vi "Initialize-parameter-refs.vi"(8 "error in (no error)":errorcluster, 11 "Data ref. in":refnum<data-value>) -> (0 "error out":errorcluster, 3 "Data ref.":refnum<data-value>)   [LabVIEW 2013, in "CameraVision.lvlib" / "CV-Main.lvclass"]
uses:
  CV-Main.lvclass
  CV-Main.lvclass/CV-Main.ctl
  Acquisition/CV-Acquisition.lvclass
  Analysis/CV-Analysis.lvclass
  Configuration/CV-Configuration.lvclass
  Correction/CV-Correction.lvclass
  Mapping/CV-Mapping.lvclass
  Storage/CV-Storage.lvclass
  Temperature/CV-Temperature.lvclass
  Filter/CV-Filter.lvclass
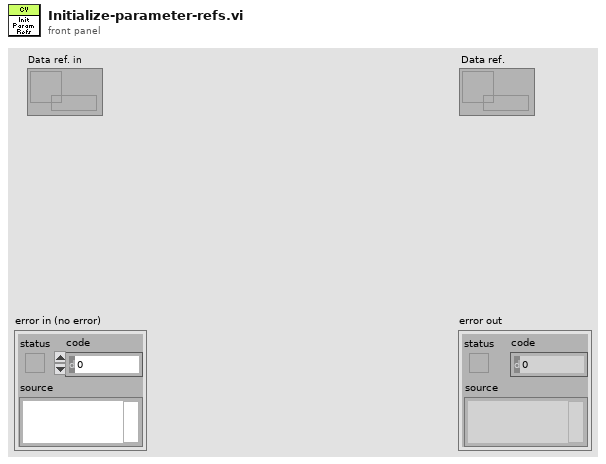
[diagram p1: front panel]
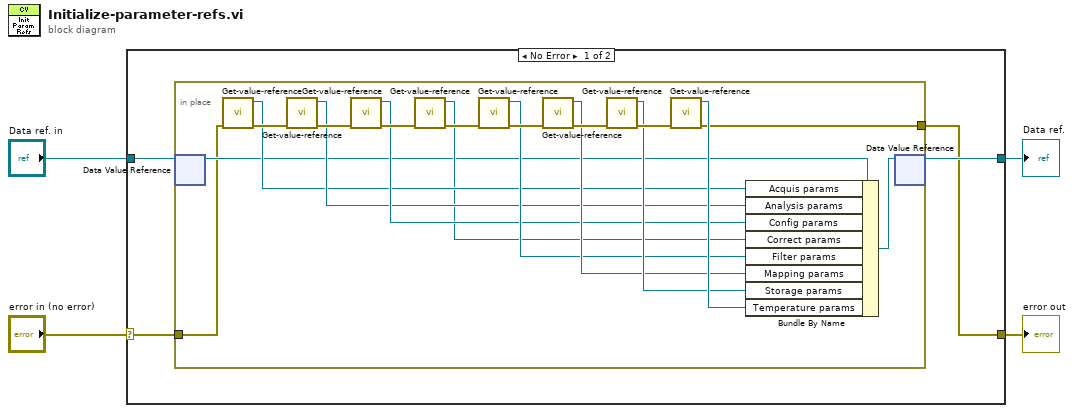
[diagram p0: block diagram]
diagram:
  n1 = case shown="No Error" "error in (no error)" {
    selector: "error in (no error)" -> [w6 w29]
    tunnel: [w5 w29] -> w3
    tunnel: "Data ref. in" -> [w8 w28]
    tunnel: [w7 w28] -> w1
    frame No Error {
      n2 = in-place {
        in-place-border: w6 -> [w10]
        in-place-border: [w9] -> w5
        n3 = in-place-dvr #1(w8) -> (w11:refnum<class "CV-Main.lvclass">)  [unwired: 1 out]
        n4 = call "Get-value-reference.vi"("error in (no error)"=w10) -> ("error out"=w27:errorcluster, "Acquis. params. ref."=w14:refnum<data-value>)  [unwired: 9 in]
        n5 = call "Get-value-reference.vi"("error in (no error)"=w27) -> ("error out"=w26:errorcluster, "Analysis params. ref."=w15:refnum<data-value>)  [unwired: 9 in]
        n6 = call "Get-value-reference.vi"("error in (no error)"=w26) -> ("error out"=w25:errorcluster, "Config. params. ref."=w16:refnum<data-value>)  [unwired: 9 in]
        n7 = call "Get-value-reference.vi"("error in (no error)"=w25) -> ("error out"=w22:errorcluster, "Correct. params. ref."=w13:refnum<data-value>)  [unwired: 9 in]
        n8 = call "Get-value-reference.vi"("error in (no error)"=w22) -> ("error out"=w21:errorcluster, "Filter params. ref."=w17:refnum<data-value>)  [unwired: 9 in]
        n9 = call "Get-value-reference.vi"("error in (no error)"=w21) -> ("error out"=w24:errorcluster, "Mapping params. ref."=w18:refnum<data-value>)  [unwired: 9 in]
        n10 = call "Get-value-reference.vi"("error in (no error)"=w24) -> ("error out"=w23:errorcluster, "Storage params. ref."=w19:refnum<data-value>)  [unwired: 9 in]
        n11 = call "Get-value-reference.vi"("error in (no error)"=w23) -> ("error out"=w9:errorcluster, "Temp. params. ref."=w20:refnum<data-value>)  [unwired: 9 in]
        n12 = Bundle By Name(cluster=w11, "Acquis params"=w14, "Analysis params"=w15, "Config params"=w16, "Correct params"=w13, "Filter params"=w17, "Mapping params"=w18, "Storage params"=w19, "Temperature params"=w20) -> (w12:refnum<class "CV-Main.lvclass">)
        n13 = in-place-dvr #1(w12) -> (w7:refnum<data-value>)  [unwired: 1 out]
      }
    }
    frame Error {
    }
  }
  "error out" <- w3
  "Data ref." <- w1
